vi "Dialogue - Two Button.vi"(9 "False Button Text (Cancel)":string="Cancel", 10 "True Button Text":string, 11 "Message":string) -> (3 "True Button Pressed":bool)   [LabVIEW 2021, in "Utility.lvlib"]
uses:
  Utility.lvlib
  <userlib>/_OpenG.lib/appcontrol/appcontrol.llb/openg_application_control.lvlib
  UI/System Button (without mouse hover).ctl
panel:
  in  "False Button":T1
  in  "True Button":T1
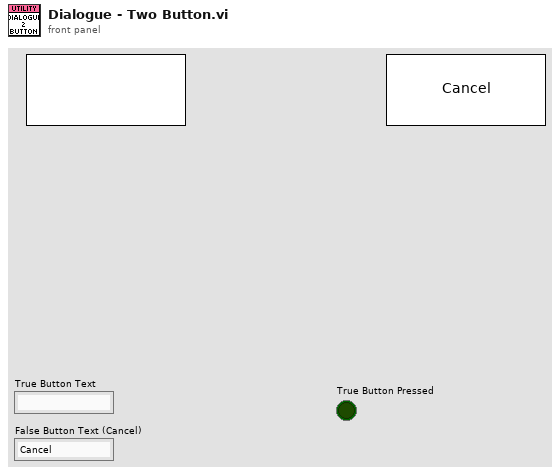
[diagram p1: front panel]
types:
  T1 = typedef "Utility.lvlib/System Button (without mouse hover).ctl" = bool
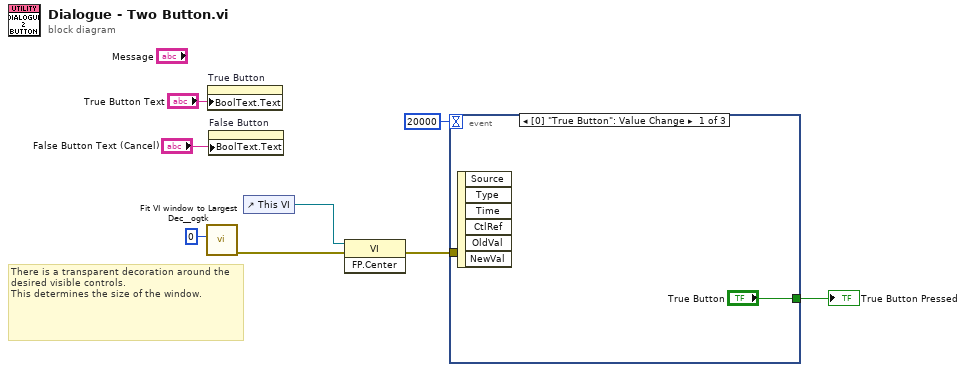
[diagram p0: block diagram]
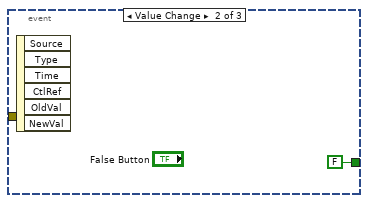
[diagram p2: hidden frame]
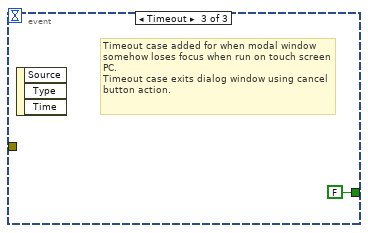
[diagram p3: hidden frame]
diagram:
  # "There is a transparent decoration around the desired visible controls.\nThis determines the size of the window."
  n1 = call <userlib>:"Fit VI window to Largest Dec__ogtk.vi"("border spacing (2 px)"=0) -> ("error out"=w3:errorcluster)  [unwired: 2 in, 4 out]
  n2 = property on="True Button" class="Bool"("BoolText.Text"="True Button Text") -> ()  [unwired: 2 in, 2 out]
  n3 = property on="False Button" class="Bool"("BoolText.Text"="False Button Text (Cancel)") -> ()  [unwired: 2 in, 2 out]
  n4 = control-ref of="This VI"() -> (w4:refnum<vi>)
  n5 = invoke class="VI" method="FP.Center"(reference=w4, error in=w3) -> (error out=w2:errorcluster)  [unwired: 1 in, 2 out]
  n6 = event shown="[0] \"True Button\": Value Change" {
    selector: _ -> [_ _ _]
    dyn-events: _ -> [_ _ _]
    timeout: 20000 -> [_ _ _]
    tunnel: w2 -> [_ _ _]
    tunnel: ["True Button" FALSE ("True Button") FALSE ("True Button")] -> w6
    event Value Change {
      n7 = event-data() -> ()  [unwired: 1 in, 6 out]
    }
    event Value Change {
      n8 = event-data() -> ()  [unwired: 1 in, 6 out]
    }
    event Timeout {
      # "Timeout case added for when modal window somehow loses focus when run on touch screen PC.\nTimeout case exits dialog window using cancel button action."
      n9 = event-data() -> ()  [unwired: 1 in, 3 out]
    }
  }
  "True Button Pressed" <- w6
